vi "Validate and Coerce Timing Window.vi"(7 "Max engine angle":dbl min=0.0 format="%#_f", 9 "Min changed last":bool, 10 "Max":dbl, 11 "Min":dbl) -> (2 "Coerced maximum":dbl, 3 "Coerced minimum":dbl)   [LabVIEW 2015, in "Engine Simulation Toolkit System Explorer.lvlib"]
uses:
  Engine Simulation Toolkit System Explorer.lvlib
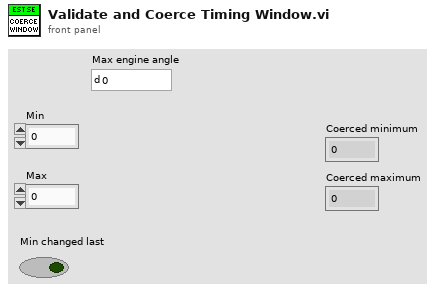
[diagram p1: front panel]
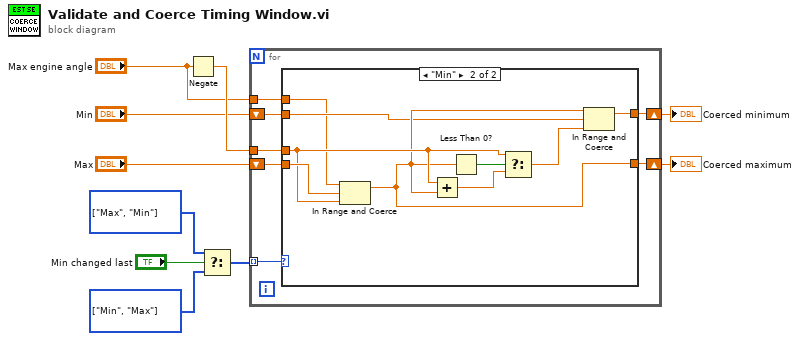
[diagram p0: block diagram]
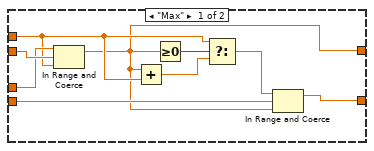
[diagram p2: hidden frame]
diagram:
  w8 = enum16{"Min", "Max"}[] [enum."Min", enum."Max"] items=["Min", "Max"]
  w9 = enum16{"Min", "Max"}[] [enum."Max", enum."Min"] items=["Min", "Max"]
  n1 = Negate(x="Max engine angle") -> (-x=w5:dbl)
  n2 = Select(t=w9, s="Min changed last", f=w8) -> (s? t:f=w7:enum16{"Min", "Max"}[])
  n3 = for {
    tunnel: w7 -> [w17] mode=indexing
    tunnel: w5 -> [w15]
    shift-right: [w14] -> w4
    shift-left: "Max" -> [w16]
    shift-right: [w12] -> w1
    shift-left: "Min" -> [w13]
    tunnel: "Max engine angle" -> [w11]
    n4 = case shown="\"Min\"" w17 {
      tunnel: w16 -> [w23 w31]
      tunnel: w15 -> [w20 w30]
      tunnel: [w22 w29] -> w14
      tunnel: w13 -> [w21 w28]
      tunnel: [w18 w33] -> w12
      tunnel: w11 -> [w19 w27]
      frame "Max" {
        n5 = In Range and Coerce(upper limit=w20, x=w21, lower limit=w19) -> (coerced(x)=w18:dbl)  [unwired: 1 out]
        n6 = Add(x=w18, y=w19) -> (x+y=w26:dbl)
        n7 = Greater Or Equal To 0?(x=w18) -> (x >= 0?=w25:bool)
        n8 = Select(t=w19, s=w25, f=w26) -> (s? t:f=w24:dbl)
        n9 = In Range and Coerce(upper limit=w24, x=w23, lower limit=w18) -> (coerced(x)=w22:dbl)  [unwired: 1 out]
      }
      frame "Min" {
        n10 = In Range and Coerce(upper limit=w27, x=w31, lower limit=w30) -> (coerced(x)=w29:dbl)  [unwired: 1 out]
        n11 = Add(x=w30, y=w29) -> (x+y=w34:dbl)
        n12 = Less Than 0?(x=w29) -> (x < 0?=w35:bool)
        n13 = Select(t=w30, s=w35, f=w34) -> (s? t:f=w32:dbl)
        n14 = In Range and Coerce(upper limit=w29, x=w28, lower limit=w32) -> (coerced(x)=w33:dbl)  [unwired: 1 out]
      }
    }
  }
  "Coerced minimum" <- w1
  "Coerced maximum" <- w4
